vi "Analysis Template.vi"() -> ()   [LabVIEW 2020]
panel:
  out "error out":errorcluster
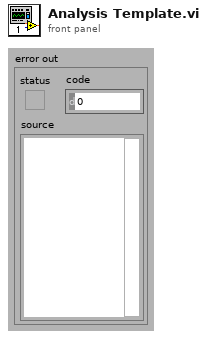
[diagram p1: front panel]
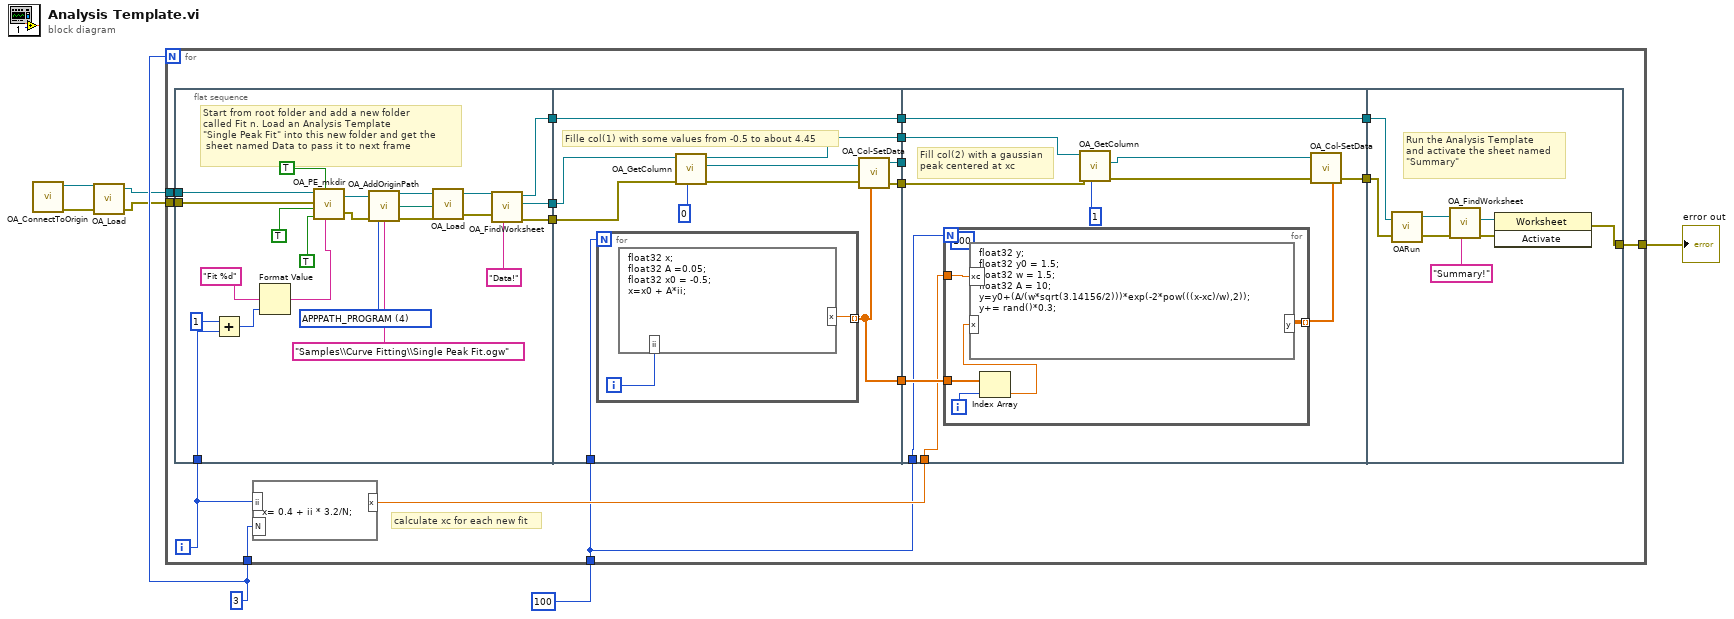
[diagram p0: block diagram]
diagram:
  w6 = 3
  n1 = call "OA_ConnectToOrigin.vi"() -> ("error out"=w3:errorcluster, "Origin.IOApplication"=w4:refnum<k7>)  [unwired: 8 in]
  n2 = call "OA_Load.vi"("error in (no error)"=w3, "Origin.IOApplication"=w4) -> ("error out"=w2:errorcluster, "Origin.IOApplication"=w1:refnum<k7>)  [unwired: 1 in, 1 out]
  n3 = for {
    N: w6 -> [_]
    tunnel: w2 -> [w19]
    tunnel: 100 -> [w12]
    tunnel: w6 -> [w11]
    tunnel: [w9] -> w5
    tunnel: w1 -> [w8]
    i -> [w10]
    # "calculate xc for each new fit"
    n4 = flat-sequence {
      tunnel: w8 -> [w27]
      tunnel: w19 -> [w26]
      tunnel: [w35] -> w18
      tunnel: [w34] -> w17
      tunnel: [w33] -> w16
      tunnel: w10 -> [w29]
      tunnel: [w55] -> w24
      tunnel: [w54] -> w23
      tunnel: [w53] -> w22
      tunnel: [w52] -> w21
      tunnel: w18 -> [w49]
      tunnel: w17 -> [w51]
      tunnel: w16 -> [w50]
      tunnel: [w49] -> w14
      tunnel: w12 -> [w48]
      tunnel: w24 -> [_]
      tunnel: w23 -> [w68]
      tunnel: w22 -> [w67]
      tunnel: w21 -> [w65]
      tunnel: [w61] -> w20
      tunnel: [w64] -> w15
      tunnel: w14 -> [w64]
      tunnel: w13 -> [w63]
      tunnel: w12 -> [w62]
      tunnel: w20 -> [w78]
      tunnel: w15 -> [w79]
      tunnel: [w77] -> w9
      frame #0 {
        w38 = 4 items=["APPPATH_USER"=2, "APPPATH_GROUP"=3, "APPPATH_PROGRAM"=4] ("Type")
        # "Start from root folder and add a new folder\ncalled Fit n. Load an Analysis Template\n\"Single Peak Fit\" into this new folder and get the \n sheet named Data to pass it to next frame"
        n5 = Add(x=1, y=w29) -> (x+y=w30:i32)
        n6 = Format Value(format string="Fit %d", value (0)=w30) -> (output string=w31:string)  [unwired: 1 in]
        n7 = call "OA_PE_mkdir.vi"("name"=w31, "from root"=TRUE, "cd"=TRUE, "use existing"=TRUE ("cd"), "Error In"=w26, "Origin.IOApplication"=w27) -> ("Error IO Out"=w37:errorcluster, "Origin.IOApplication Out"=w36:refnum<k7>)
        n8 = call "OA_AddOriginPath.vi"("Origin.IOApplication"=w36, "error in (no error)"=w37, "Type"=w38, "Filename"="Samples\\Curve Fitting\\Single Peak Fit.ogw") -> ("Origin.IOApplication"=w41:refnum<k7>, "path out"=w42:path, "error out"=w40:errorcluster)  [unwired: 9 in]
        n9 = call "OA_Load.vi"("error in (no error)"=w40, "Path"=w42, "Origin.IOApplication"=w41) -> ("error out"=w45:errorcluster, "Origin.IOApplication"=w44:refnum<k7>)  [unwired: 1 out]
        n10 = call "OA_FindWorksheet.vi"("Name"="Data!", "error in (no error)"=w45, "Origin.IOApplication"=w44) -> ("error out"=w33:errorcluster, "Origin.Worksheet"=w34:refnum<k7>, "Origin.IOApplication"=w35:refnum<k7>)  [unwired: 6 in]
      }
      frame #1 {
        # "Fille col(1) with some values from -0.5 to about 4.45"
        n11 = for {
          N: w48 -> [_]
          tunnel: [w59] -> w52 mode=indexing
          i -> [w60]
          n12 = formula code="float32 x; \nfloat32 A =0.05;\nfloat32 x0 = -0.5;\nx=x0 + A*ii;"("ii"=w60) -> ("x"=w59:sgl)
        }
        n13 = call "OA_GetColumn.vi"("Column Name/Index"=0 ("nOffset"), "error in (no error)"=w50, "Origin.Worksheet"=w51) -> ("error out"=w58:errorcluster, "Origin.Column"=w57:refnum<k7>, "Origin.Worksheet"=w53:refnum<k7>)  [unwired: 6 in]
        n14 = call "OA_Col-SetData.vi"("Origin.Column"=w57, "error in (no error)"=w58, "data"=w52) -> ("Origin.Column Out"=w55:refnum<k7>, "error out"=w54:errorcluster)  [unwired: 4 in, 1 out]
      }
      frame #2 {
        (unwired) 100
        # "Fill col(2) with a gaussian\npeak centered at xc"
        n15 = for {
          N: w62 -> [_]
          tunnel: [w76] -> w66 mode=indexing
          tunnel: w65 -> [w74]
          tunnel: w63 -> [w72]
          i -> [w75]
          n16 = Index Array(array=w74, index=w75) -> (element=w73:sgl)
          n17 = formula code="float32 y; \nfloat32 y0 = 1.5;\nfloat32 w = 1.5;\nfloat32 A = 10;\ny=y0+(A/(w*sqrt(3.14156/2)))*exp(-2*pow(((x-xc)/w),2));\ny+= rand()*0.3;"("x"=w73, "xc"=w72) -> ("y"=w76:sgl)
        }
        n18 = call "OA_GetColumn.vi"("Column Name/Index"=1 ("nOffset"), "error in (no error)"=w68, "Origin.Worksheet"=w67) -> ("error out"=w71:errorcluster, "Origin.Column"=w70:refnum<k7>)  [unwired: 6 in, 1 out]
        n19 = call "OA_Col-SetData.vi"("Origin.Column"=w70, "error in (no error)"=w71, "data"=w66) -> ("error out"=w61:errorcluster)  [unwired: 4 in, 2 out]
      }
      frame #3 {
        # "Run the Analysis Template\nand activate the sheet named \n\"Summary\""
        n20 = call "OARun.vi"("Origin.IOApplication"=w79, "Error IO"=w78) -> ("Origin.IOApplication"=w81:refnum<k7>, "Error IO Out"=w82:errorcluster)  [unwired: 1 out]
        n21 = call "OA_FindWorksheet.vi"("Name"="Summary!", "error in (no error)"=w82, "Origin.IOApplication"=w81) -> ("error out"=w84:errorcluster, "Origin.Worksheet"=w83:refnum<k7>)  [unwired: 6 in, 1 out]
        n22 = invoke class="Worksheet" method="Activate"(reference=w83, error in=w84) -> (error out=w77:errorcluster)  [unwired: 1 in, 2 out]
      }
    }
    n23 = formula code="x= 0.4 + ii * 3.2/N;"("ii"=w10, "N"=w11) -> ("x"=w13:dbl)
  }
  "error out" <- w5
